vi "create_stim_array.vi"(8 "error in":errorcluster, 11 "Stim protocol":T1={"Frequency"=0.01, "Pulse duration"=0.001, "Stop after"=0.0} {"Stop after" min=0.0 max=500.0; "Pulse duration" min=0.001 max=0.1; "Frequency" min=0.01 max=200.0 step=1.0}) -> (0 "error out":errorcluster, 3 "Stim array":dbl[](array[numeric]))   [LabVIEW 2010]
uses:
  ChR2Stimulator_RK110722/typedefs/stim_protocol_cluster.ctl
panel:
  # "0 for manual stop"
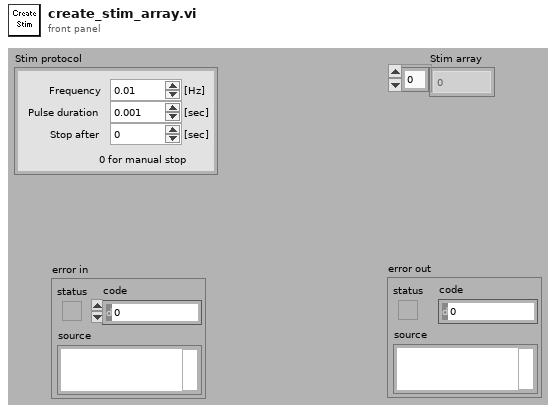
[diagram p1: front panel]
types:
  T1 = typedef "stim_protocol_cluster.ctl" = cluster{"Frequency":dbl, "Pulse duration":dbl, "Stop after":dbl}
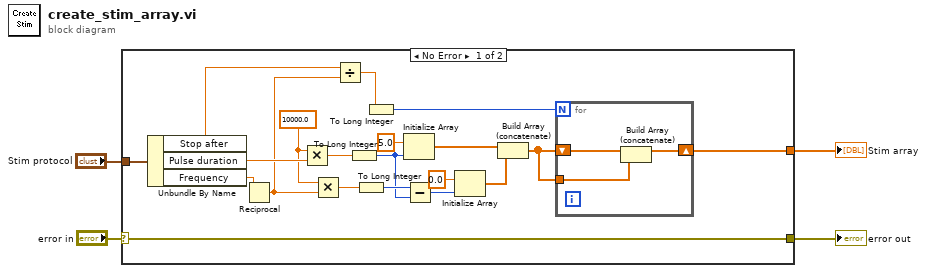
[diagram p0: block diagram]
diagram:
  n1 = case shown="No Error" "error in" {
    selector: "error in" -> [w24 w28]
    tunnel: [w24 w28] -> w3
    tunnel: "Stim protocol" -> [w23 _]
    tunnel: [w5 _] -> w1
    frame No Error {
      w18 = 10000.0 ("x")
      n2 = Unbundle By Name(w23) -> ("Stop after"=w10:dbl, "Pulse duration"=w22:dbl, "Frequency"=w19:dbl)
      n3 = Reciprocal(x=w19) -> (1/x=w9:dbl)
      n4 = Multiply(x=w18, y=w22) -> (x*y=w21:dbl)
      n5 = Multiply(x=w18, y=w9) -> (x*y=w17:dbl)
      n6 = Divide(x=w10, y=w9) -> (x/y=w8:dbl)
      n7 = To Long Integer(number=w21) -> (32bit integer=w15:i32)
      n8 = To Long Integer(number=w17) -> (32bit integer=w16:i32)
      n9 = To Long Integer(number=w8) -> (32bit integer=w7:i32)
      n10 = Initialize Array(5.0 ("element"), w15) -> (w12:dbl[])
      n11 = Subtract(x=w16, y=w15) -> (x-y=w14:i32)
      n12 = Initialize Array(0.0 ("element"), w14) -> (w11:dbl[])
      n13 = Build Array (concatenate)(w12, w11) -> (w6:dbl[])
      n14 = for {
        N: w7 -> [_]
        shift-right: [w25] -> w5
        shift-left: w6 -> [w27]
        tunnel: w6 -> [w26]
        n15 = Build Array (concatenate)(w27, w26) -> (w25:dbl[])
      }
    }
    frame Error {
    }
  }
  "error out" <- w3
  "Stim array" <- w1
